vi "execute.vi"(8 "error in (no error)":errorcluster, 10 "ComponentData.lvclass":refnum<class "ComponentData.lvclass">, 11 "BusyState in":refnum<class "DisabledState.lvclass">) -> (0 "error out":errorcluster, 2 "ComponentData.lvclass 2":refnum<class "ComponentData.lvclass">, 3 "BusyState out":refnum<class "DisabledState.lvclass">)   [LabVIEW 2013, in "ComponentData.lvlib" / "DisabledState.lvclass"]
uses:
  <userlib>/Common/Component/common_application/RT/ComponentData/ComponentState/DisabledState/DisabledState.lvclass
  <userlib>/Common/Component/common_application/RT/ComponentData/ComponentData/ComponentData.lvclass
  <userlib>/Common/Component/common_application/RT/ComponentData/ComponentState/ComponentState/ComponentState.lvclass
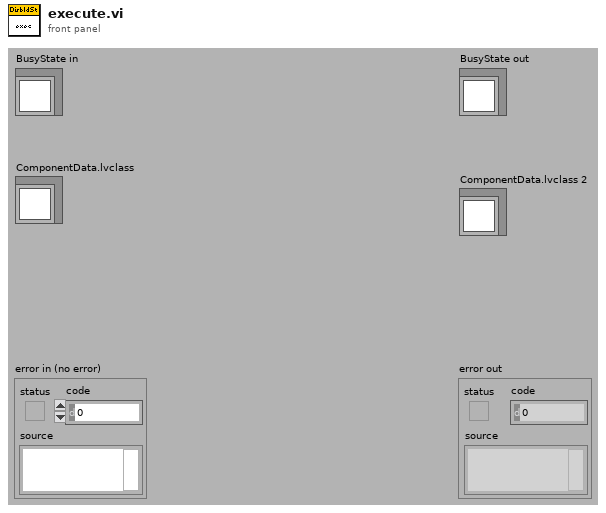
[diagram p1: front panel]
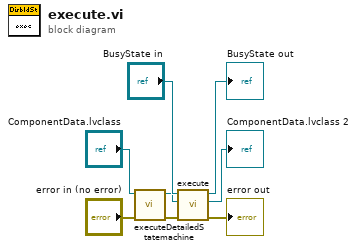
[diagram p0: block diagram]
diagram:
  n1 = call-dynamic "executeDetailedStatemachine.vi"("error in (no error)"="error in (no error)", "ComponentData in"="ComponentData.lvclass") -> ("error out"=w1:errorcluster, "ComponentData out"=w3:refnum<class "ComponentData.lvclass">)  [unwired: 8 in]
  n2 = call-parent "execute.vi"("error in (no error)"=w1, "ComponentData.lvclass"=w3, "ComponentState in"="BusyState in") -> ("error out"=→"error out":errorcluster, "ComponentData.lvclass 2"=→"ComponentData.lvclass 2":refnum<class "ComponentData.lvclass">, "ComponentState out"=→"BusyState out":refnum<class "DisabledState.lvclass">)  [unwired: 6 in]
